vi "Router - Globals.vi"() -> ()   [LabVIEW 2016, in "PXImc Router.lvlib"]
uses:
  PXImc Router.lvlib
panel:
  out "Stop":bool
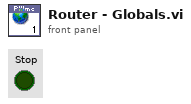
[diagram p1: front panel]
diagram:
